vi "Config.Get Name of exe.vi"(8 "error in (no error)":errorcluster) -> (0 "error out":errorcluster, 2 "Path":path)   [LabVIEW 2018]
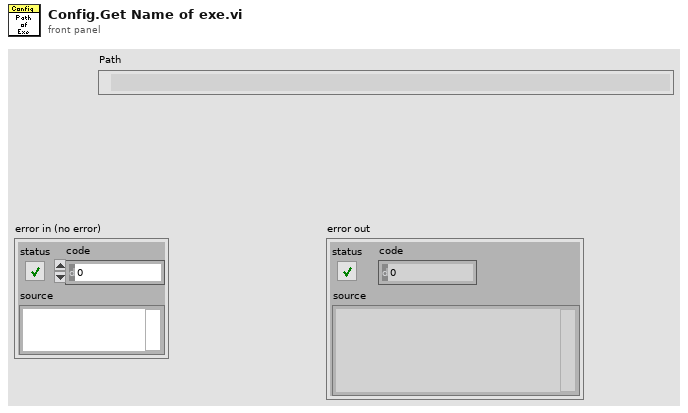
[diagram p1: front panel]
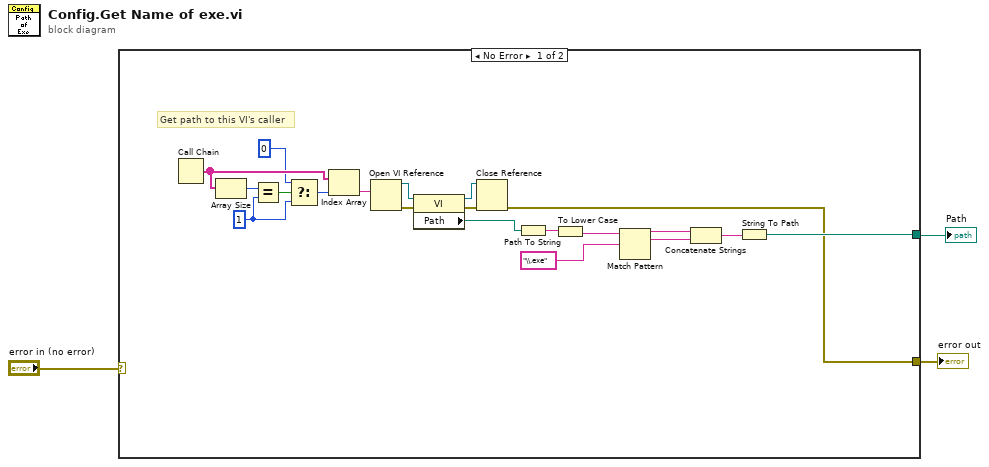
[diagram p0: block diagram]
diagram:
  n1 = case shown="No Error" "error in (no error)" {
    selector: "error in (no error)" -> [_ w24]
    tunnel: [w4 w24] -> w2
    tunnel: [w5 _] -> w1
    frame No Error {
      w19 = 1 ("index")
      # "Get path to this VI's caller"
      n2 = Call Chain() -> (call chain=w23:string[])
      n3 = Array Size(array=w23) -> (size(s)=w20:i32)
      n4 = Equal?(x=w20, y=w19) -> (x = y?=w22:bool)
      n5 = Select(t=0, s=w22, f=w19) -> (s? t:f=w21:i32)
      n6 = Index Array(array=w23, index=w21) -> (element=w15:string)
      n7 = Open VI Reference(vi path=w15) -> (vi reference=w16:refnum<vi>, error out=w17:errorcluster)  [unwired: 5 in]
      n8 = property class="VI"(reference=w16, error in=w17) -> (reference out=w13:refnum<vi>, error out=w14:errorcluster, "Path"=w12:path)
      n9 = Close Reference(reference=w13, error in (no error)=w14) -> (error out=w4:errorcluster)
      n10 = Path To String(path=w12) -> (string=w11:string)
      n11 = To Lower Case(string=w11) -> (all lower case string=w10:string)
      n12 = Match Pattern(string=w10, regular expression="\\.exe") -> (before substring=w8:string, match substring=w7:string)  [unwired: 1 in, 2 out]
      n13 = Concatenate Strings(w8, w7) -> (w6:string)
      n14 = String To Path(string=w6) -> (path=w5:path)
    }
    frame Error {
    }
  }
  "error out" <- w2
  "Path" <- w1
